vi "Launch Async force control value.vi"   [LabVIEW 2021]
uses:
  Options.ctl
types:
  T1 = enum32{"Invalid", "Standard", "Closed", "Hidden", "Minimized", "Maximized"}
  T2 = typedef "Options.ctl" = u16
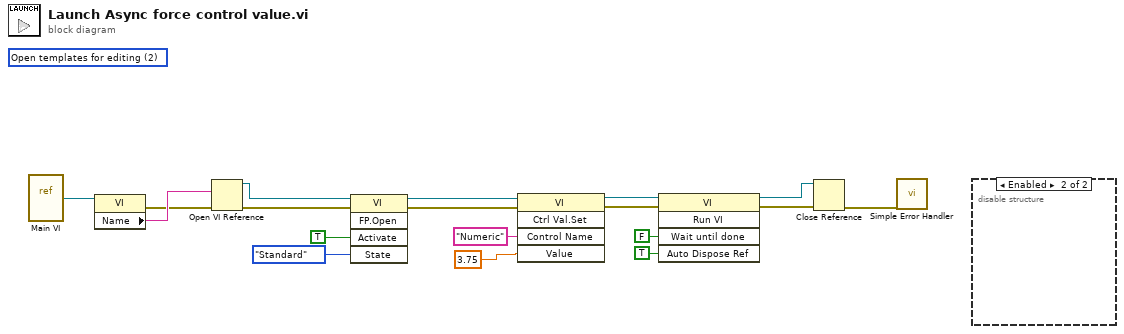
[diagram p0: block diagram]
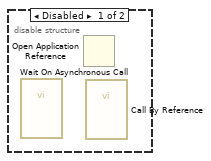
[diagram p2: hidden frame]
diagram:
  (unwired) T2 2 items=["Record modifications"=1, "Open templates for editing"=2] ("Ring")
  n1 = vi-ref "Main VI.vi"() -> (w17:refnum<vi>)
  n2 = property class="VI"(reference=w17) -> (error out=w15:errorcluster, "Name"=w16:string)  [unwired: 1 in, 1 out]
  n3 = Open VI Reference(vi path=w16, error in (no error)=w15) -> (vi reference=w9:refnum<vi>, error out=w14:errorcluster)  [unwired: 4 in]
  n4 = invoke class="VI" method="FP.Open"(reference=w9, error in=w14, "Activate"=TRUE ("Activate?"), "State"=T1."Standard") -> (reference out=w8:refnum<vi>, error out=w10:errorcluster)  [unwired: 1 in, 3 out]
  n5 = invoke class="VI" method="Ctrl Val.Set"(reference=w8, error in=w10, "Control Name"="Numeric", "Value"=3.75) -> (reference out=w4:refnum<vi>, error out=w13:errorcluster)  [unwired: 1 in, 3 out]
  n6 = invoke class="VI" method="Run VI"(reference=w4, error in=w13, "Wait until done"=FALSE ("Wait Until Done"), "Auto Dispose Ref"=TRUE ("Auto Dispose Reference")) -> (reference out=w3:refnum<vi>, error out=w5:errorcluster)  [unwired: 1 in, 3 out]
  n7 = Close Reference(reference=w3, error in (no error)=w5) -> (error out=w18:errorcluster)
  n8 = call <vilib>:"Simple Error Handler.vi"("error in (no error)"=w18) -> ()  [unwired: 4 in, 5 out]
  n9 = disable-structure shown="Enabled" {
    frame Disabled {
      n10 = call-by-ref "Wait On Asynchronous Call"() -> ()  [unwired: 2 in, 2 out]
      n11 = Open Application Reference() -> ()  [unwired: 4 in, 2 out]
      n12 = call-by-ref "?"() -> ()  [unwired: 2 in, 2 out]
    }
    frame Enabled {
    }
  }
